vi "Server.vi"() -> ()   [LabVIEW 2020]
panel:
  in  "stop":bool
  out "error out":errorcluster
  in  "data in":string
  out "String":string
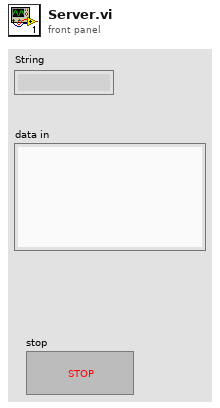
[diagram p1: front panel]
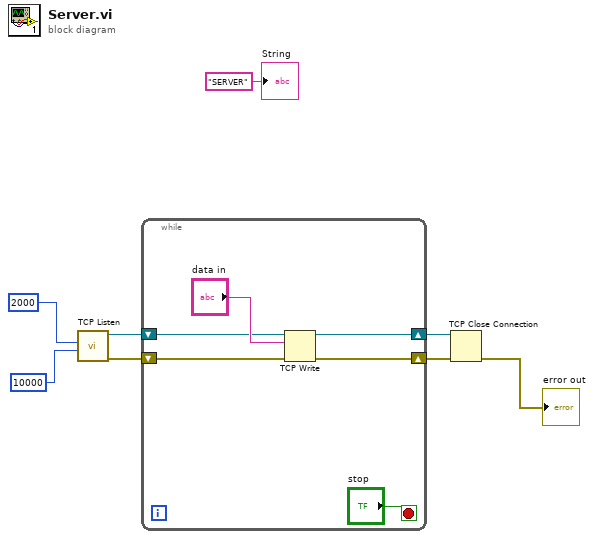
[diagram p0: block diagram]
diagram:
  n1 = call <vilib>:"TCP Listen.vi"("timeout ms (wait forever: -1)"=10000, "port"=u16 2000) -> ("error out"=w2:errorcluster, "connection ID"=w5:refnum<k5>)  [unwired: 5 in, 3 out]
  n2 = while {
    shift-right: [w13] -> w6
    shift-left: w5 -> [w12]
    shift-right: [w10] -> w1
    shift-left: w2 -> [w11]
    stop <- "stop" stop-if-true
    n3 = TCP Write(connection ID=w12, data in="data in", error in (no error)=w11) -> (connection ID out=w13:refnum<k5>, error out=w10:errorcluster)  [unwired: 1 in, 1 out]
  }
  n4 = TCP Close Connection(connection ID=w6, error in (no error)=w1) -> (error out=→"error out":errorcluster)  [unwired: 1 in, 1 out]
  "String" <- "SERVER" ("String")
